vi "CM-TDT-Unregister Events.vi"(9 "Lists":cluster{"AO":T2, "AI":T2, "DO":T2, "DI":T2}, 10 "Tables":cluster{"AO":T1, "AI":T1, "DO":T1, "DI":T1}, 11 "Event Registration Refnum":refnum<event-registration>) -> ()   [LabVIEW 2020]
uses:
  Utility VIs/Controls/KListboxEx/Events.ctl
  Utility VIs/Controls/KListboxEx/Event Action.ctl
  Utility VIs/Controls/KTable/Events.ctl
  Utility VIs/Controls/KTable/Event Data.ctl
  Utility VIs/Controls/KTable/Event Type.ctl
  Utility VIs/Controls/KListboxEx/KListboxEx.xctl
  Utility VIs/Controls/KTable/KTable.xctl
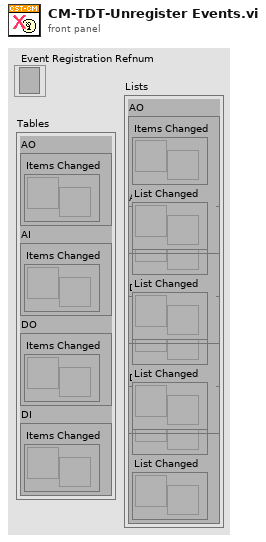
[diagram p1: front panel]
types:
  T1 = typedef "KTable.xctl/Events.ctl" = cluster{"Items Changed":refnum<user-event>}
  T2 = typedef "KListboxEx.xctl/Events.ctl" = cluster{"Items Changed":refnum<user-event>, "List Changed":refnum<user-event>}
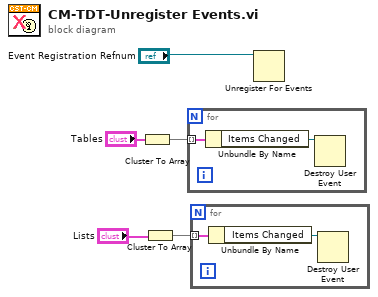
[diagram p0: block diagram]
diagram:
  n1 = Cluster To Array(cluster="Tables") -> (array=w2:T1[])
  n2 = Cluster To Array(cluster="Lists") -> (array=w1:T2[])
  n3 = for {
    tunnel: w2 -> [w7] mode=indexing
    n4 = Unbundle By Name(w7) -> ("Items Changed"=w6:refnum<user-event>)
    n5 = Destroy User Event(user event=w6) -> ()  [unwired: 1 in, 1 out]
  }
  n6 = for {
    tunnel: w1 -> [w9] mode=indexing
    n7 = Unbundle By Name(w9) -> ("Items Changed"=w8:refnum<user-event>)
    n8 = Destroy User Event(user event=w8) -> ()  [unwired: 1 in, 1 out]
  }
  n9 = Unregister For Events(event registration refnum="Event Registration Refnum") -> ()  [unwired: 1 in, 1 out]
